vi "create data file header.vi"(11 "fileIO":T1) -> (3 "header string":string)   [LabVIEW 2018]
uses:
  type defs/file IO data.ctl
  type defs/channelControl.ctl
  RT/Type Defs/channelScalingTypes.ctl
  RT/Type Defs/scalingMethods.ctl
  Github/ICL-LabVIEW_General/data channels/parent class/Data Channel.lvclass
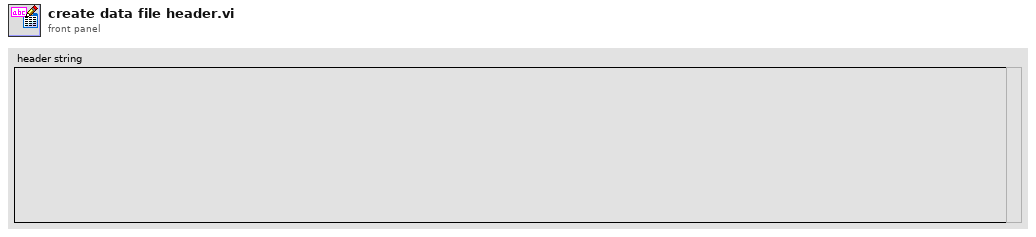
[diagram p1: front panel]
types:
  T1 = typedef "file IO data.ctl" = cluster{"params":cluster{"startFolder":path, "channelConfigPath":path}, "vars":cluster{"channelConfig ":T2[], "writing":cluster{"streaming":bool, "fixedLength":bool, "pointCount":u32, "timeZero":dbl, "pointsWritten":u32, "dataRate":u16}, "channelCount":u16, "fileTarget":cluster{"Save folder":path, "Target filename":string, "file ref":refnum<file>, "pulsatorSpeed":string, "motorSpeed":string, "valvePosition":string, "torqueFilter":bool, "pulsatorRunning":bool, "motorRunning":bool}, "channels":refnum<class "Data Channel.lvclass">[]}}
  T2 = typedef "channelControl.ctl" = cluster{"index":u16, "active":bool, "channelType":T3, "module":u16, "terminal":u16, "channelName":string, "scalingMethod":T4, "scalingParameters":dbl[], "scaledUnits":string, "tempOffset":dbl}
  T3 = typedef "channelScalingTypes.ctl" = enum16{"calculation", "measurement", "scanivalve", "output", "digital"}
  T4 = typedef "scalingMethods.ctl" = enum16{"none", "linear", "thermocouple", "polynomial", "encoder", "RTD"}
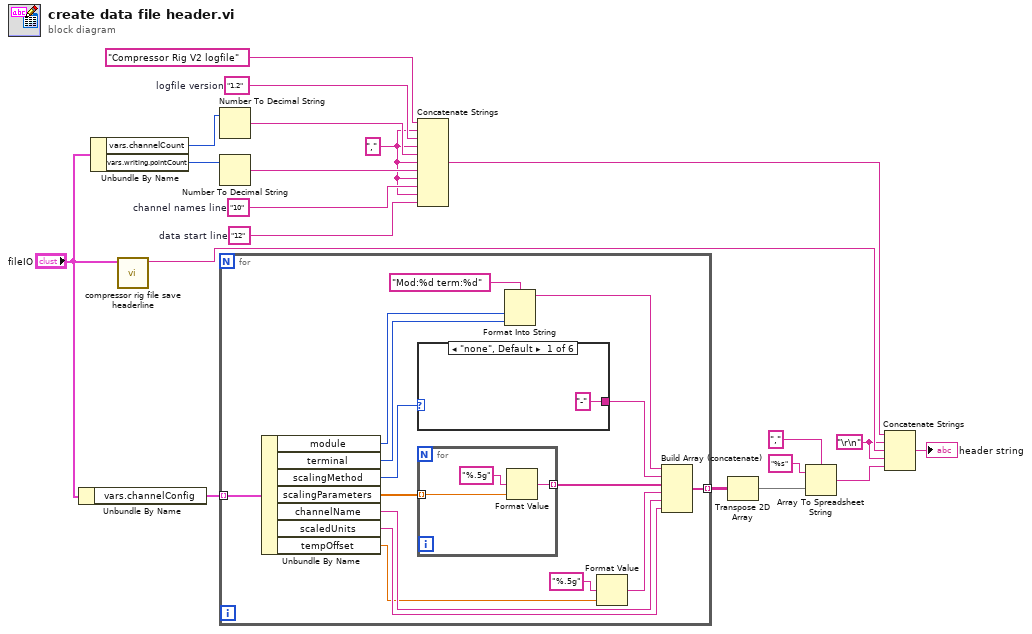
[diagram p0: block diagram]
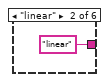
[diagram p2: hidden frame]
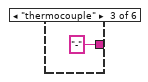
[diagram p3: hidden frame]
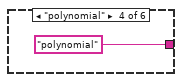
[diagram p4: hidden frame]
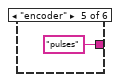
[diagram p5: hidden frame]
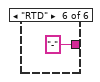
[diagram p6: hidden frame]
diagram:
  w4 = "12"  # data start line
  w6 = "10"  # channel names line
  w11 = "1.2"  # logfile version
  w5 = "," ("string")
  w16 = "\r\n"
  n1 = Unbundle By Name("fileIO") -> ("vars.channelConfig"=w13:T2[])
  n2 = Unbundle By Name("fileIO") -> ("vars.channelCount"=w9:u16, "vars.writing.pointCount"=w8:u32)
  n3 = call "compressor rig file save headerline.vi"("fileIO"="fileIO") -> ("compressorRig save file headerline"=w17:string)  [unwired: 10 in]
  n4 = Number To Decimal String(number=w9) -> (decimal integer string=w10:string)  [unwired: 1 in]
  n5 = Number To Decimal String(number=w8) -> (decimal integer string=w7:string)  [unwired: 1 in]
  n6 = for {
    tunnel: w13 -> [w35] mode=indexing
    tunnel: [w33] -> w1 mode=indexing
    n7 = Unbundle By Name(w35) -> ("module"=w26:u16, "terminal"=w25:u16, "scalingMethod"=w32:T4, "scalingParameters"=w34:dbl[], "channelName"=w28:string, "scaledUnits"=w29:string, "tempOffset"=w23:dbl)
    n8 = case shown="\"none\", Default" w32 {
      tunnel: ["-" "linear" "-" "polynomial" "pulses" "-"] -> w31
      frame "none", Default {
      }
      frame "linear" {
      }
      frame "thermocouple" {
      }
      frame "polynomial" {
      }
      frame "encoder" {
      }
      frame "RTD" {
      }
    }
    n9 = for {
      tunnel: w34 -> [w44] mode=indexing
      tunnel: [w42] -> w30 mode=indexing
      n10 = Format Value(format string="%.5g", value (0)=w44) -> (output string=w42:string)  [unwired: 1 in]
    }
    n11 = Format Into String(format string="Mod:%d term:%d", w26, w25) -> (resulting string=w24:string)  [unwired: 2 in, 1 out]
    n12 = Format Value(format string="%.5g", value (0)=w23) -> (output string=w21:string)  [unwired: 1 in]
    n13 = Build Array (concatenate)(w24, w31, w30, w21, w28, w29) -> (w33:string[])
  }
  n14 = Concatenate Strings("Compressor Rig V2 logfile" ("delimiter (Tab)"), w5, w11, w5, w10, w5, w7, w5, w6, w5, w4) -> (w3:string)
  n15 = Transpose 2D Array(2D array=w1) -> (transposed array=w18:string[][])
  n16 = Array To Spreadsheet String(delimiter (Tab)=",", array=w18, 3:"%s" ("format string")) -> (spreadsheet string=w15:string)
  n17 = Concatenate Strings(w3, w16, w17, w16, w15) -> (→"header string":string)
